vi "Delete Table.vi"() -> ()   [LabVIEW 2016, in "LV-Data.PGSQL.lvclass"]
uses:
  LV-Data.PGSQL.lvclass
panel:
  in  "Table Path":string
  out "LV-Data.PGSQL out":refnum<class "LV-Data.PGSQL.lvclass">
  out "error out":errorcluster
  in  "LV-Data.PGSQL":refnum<class "LV-Data.PGSQL.lvclass">
  in  "error in":errorcluster
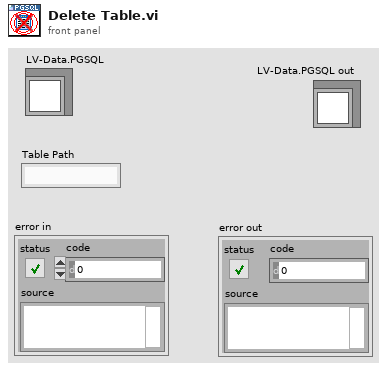
[diagram p1: front panel]
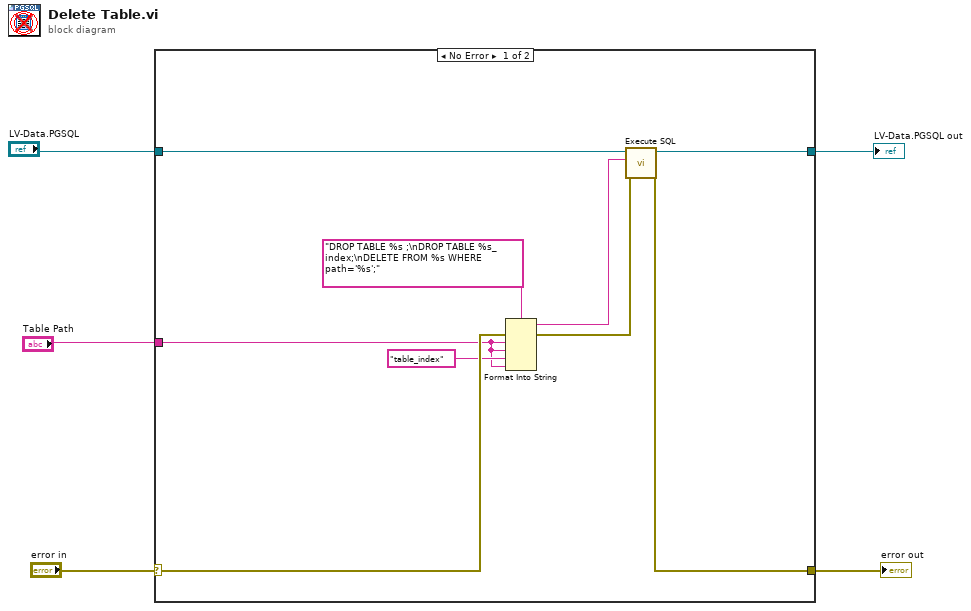
[diagram p0: block diagram]
diagram:
  n1 = case shown="No Error" "error in" {
    selector: "error in" -> [w11 w16]
    tunnel: "LV-Data.PGSQL" -> [w10 w15]
    tunnel: [w9 w16] -> w3
    tunnel: [w8 w15] -> w2
    tunnel: "Table Path" -> [w6 _]
    frame No Error {
      n2 = Format Into String(format string="DROP TABLE %s ;\nDROP TABLE %s_index;\nDELETE FROM %s WHERE path='%s';", error in=w11, w6, w6, "table_index" ("input 3"), w6) -> (resulting string=w13:string, error out=w12:errorcluster)  [unwired: 1 in]
      n3 = call "Execute SQL.vi"("error in"=w12, "SQL"=w13, "LV-Data.PGSQL"=w10) -> ("error out"=w9:errorcluster, "LV-Data.PGSQL out"=w8:refnum<class "LV-Data.PGSQL.lvclass">)  [unwired: 6 in, 1 out]
    }
    frame Error {
    }
  }
  "error out" <- w3
  "LV-Data.PGSQL out" <- w2
